vi "Clear Buffer.vi"(8 "error in (no error)":errorcluster, 11 "Ring buffer DVR":refnum<data-value>) -> (0 "error out":errorcluster)   [LabVIEW 2021, in "Ring Buffer Time Series Data.lvlib"]
uses:
  Ring Buffer Time Series Data.lvlib
  SubVIs/DVR data.ctl
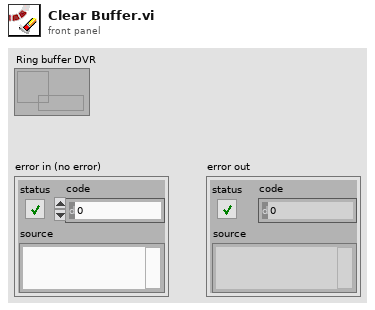
[diagram p1: front panel]
types:
  T1 = typedef "Ring Buffer Time Series Data.lvlib/DVR data.ctl" = cluster{"Timestamps":u64[], "Values":u8[], "#bytes per timestamp":i32, "Index":i32, "Size (#timestamps)":i32, "Full?":bool}
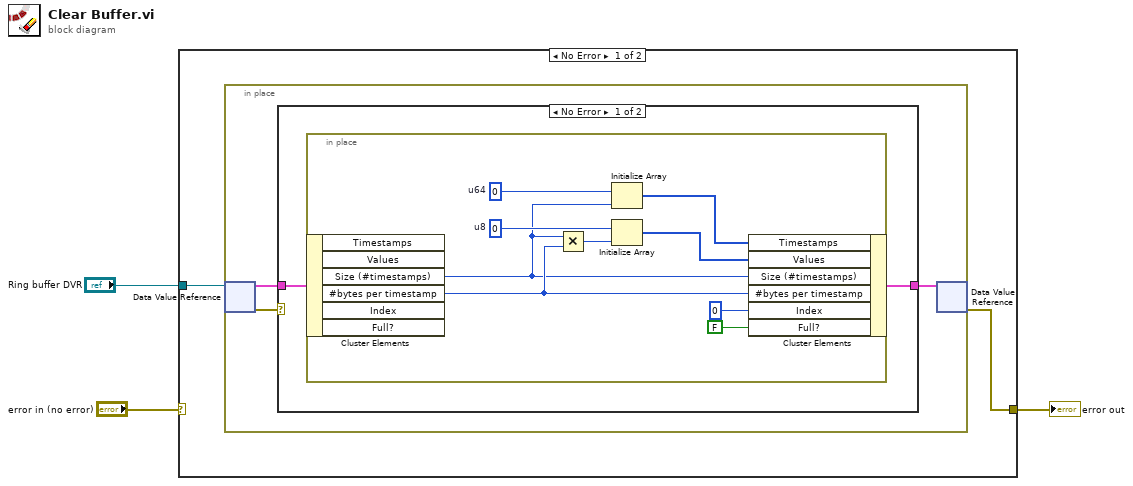
[diagram p0: block diagram]
diagram:
  n1 = case shown="No Error" "error in (no error)" {
    selector: "error in (no error)" -> [_ w21]
    tunnel: "Ring buffer DVR" -> [w5 _]
    tunnel: [w4 w21] -> w1
    frame No Error {
      n2 = in-place {
        n3 = in-place-dvr #1(w5) -> (w7:T1, w8:errorcluster)
        n4 = case shown="No Error" w8 {
          tunnel: w7 -> [w10 w20]
          tunnel: [w9 w20] -> w6
          frame No Error {
            n5 = in-place {
              w18 = u64 0  # u64
              w19 = u8 0  # u8
              n6 = in-place-cluster #2(w10) -> ("Size (#timestamps)"=w11:i32, "#bytes per timestamp"=w12:i32)  [unwired: 4 out]
              n7 = Multiply(x=w11, y=w12) -> (x*y=w17:i32)
              n8 = Initialize Array(w18, w11) -> (w16:u64[])
              n9 = Initialize Array(w19, w17) -> (w15:u8[])
              n10 = in-place-cluster #2("Timestamps"=w16, "Values"=w15, "Size (#timestamps)"=w11, "#bytes per timestamp"=w12, "Index"=0 ("data size"), "Full?"=FALSE) -> (w9:T1)
            }
          }
          frame Error {
          }
        }
        n11 = in-place-dvr #1(w6) -> (w4:errorcluster)  [unwired: 1 out]
      }
    }
    frame Error {
    }
  }
  "error out" <- w1
